vi "UTILITY Semaphore Destroy Local.vi"(3 "Semiphore":T1, 4 "Local?":bool, 5 "error in (no error)":errorcluster) -> (19 "error out":errorcluster)   [LabVIEW 2016]
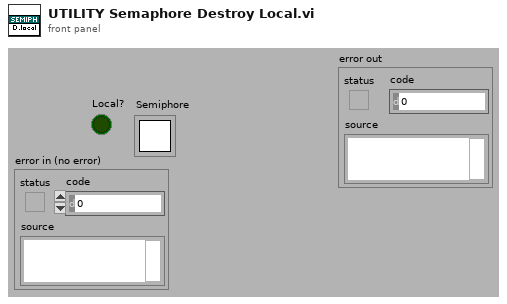
[diagram p1: front panel]
types:
  T1 = typedef "Semaphore RefNum" = refnum<k1>
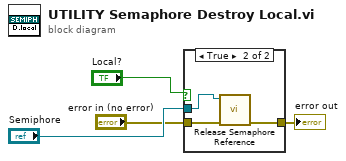
[diagram p0: block diagram]
diagram:
  n1 = case shown="True" "Local?" {
    tunnel: "error in (no error)" -> [w5 w8]
    tunnel: [w5 w7] -> w1
    tunnel: "Semiphore" -> [_ w6]
    frame False {
    }
    frame True {
      n2 = call <vilib>:"Release Semaphore Reference.vi"("error in (no error)"=w8, "semaphore"=w6) -> ("error out"=w7:errorcluster)  [unwired: 8 in, 1 out]
    }
  }
  "error out" <- w1
